vi "subDAQ1 (SubVI).vi"(3 "Sample Rate":dbl=1000.0, 4 "Number of Samples in":i32=1000) -> (0 "error out":errorcluster, 1 "Refnum out":refnum<k21>)   [LabVIEW 2018]
uses:
  <vilib>/DAQmx/create/channels.llb/DAQmx Create Channel (AI-Voltage-Basic).vi
  <vilib>/DAQmx/configure/timing.llb/DAQmx Timing (Sample Clock).vi
  <resource>/objmgr/daqmx.rc
panel:
  in  "Terminal Configuration":i32(ring)=-1 items=["default"=-1, "RSE"=10083, "NRSE"=10078, "Differential"=10106, "Pseudodifferential"=12529]
  in  "Physical Channel":tag="PXIe_NI6341/ai0"
  in  "Min Voltage":dbl=-10.0
  in  "Max Voltage":dbl=10.0
  out "Number of Samples out":i32=1000
  in  "Sample Clock Source":tag="OnboardClock"
  out "Actual Sample Rate":dbl=1000.0 format="%0.2f"
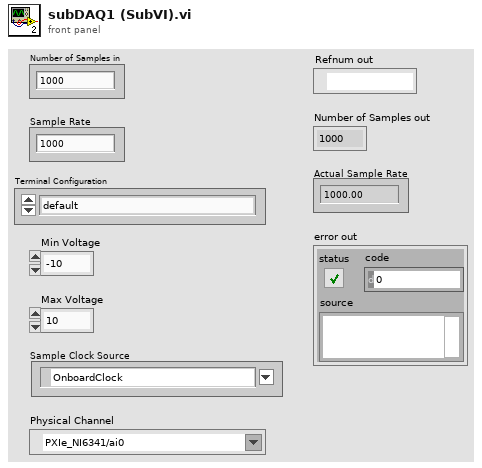
[diagram p1: front panel]
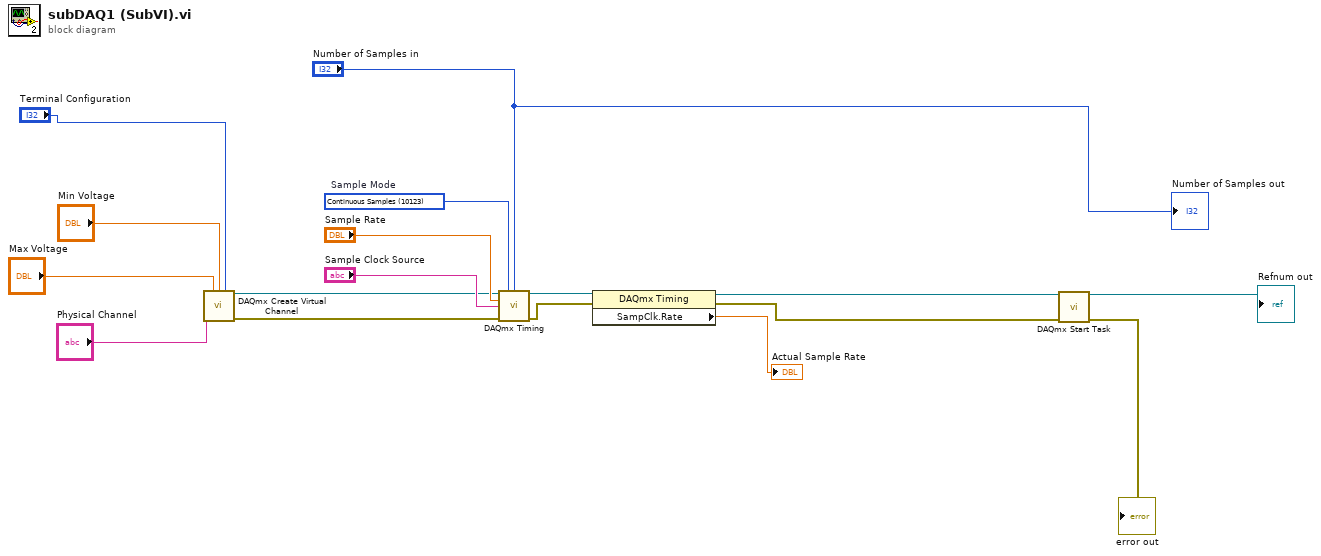
[diagram p0: block diagram]
diagram:
  w4 = 10123 items=["Finite Samples"=10178, "Continuous Samples"=10123, "Hardware Timed Single Point"=12522]  # Sample Mode
  n1 = call-poly <vilib>:"DAQmx Create Virtual Channel.vi"("maximum value"="Max Voltage", "minimum value"="Min Voltage", "input terminal configuration"="Terminal Configuration", "physical channels"="Physical Channel") -> ("task out"=w6:refnum<k21>, "error out"=w5:errorcluster)  [unwired: 10 in]
  n2 = call-poly <vilib>:"DAQmx Timing.vi"("task/channels in"=w6, "sample mode"=w4, "samples per channel"="Number of Samples in", "rate"="Sample Rate", "source"="Sample Clock Source", "error in"=w5) -> ("task out"=w2:refnum<k21>, "error out"=w3:errorcluster)  [unwired: 8 in]
  n3 = property class="DAQmx Timing"(reference=w2, error in=w3) -> (reference out=w15:refnum<k21>, error out=w16:errorcluster, "SampClk.Rate"=→"Actual Sample Rate":dbl)
  n4 = call <vilib>:"DAQmx Start Task.vi"("task/channels in"=w15, "error in"=w16) -> ("task out"=→"Refnum out":refnum<k21>, "error out"=→"error out":errorcluster)  [unwired: 12 in]
  "Number of Samples out" <- "Number of Samples in"
